vi "_folderExistOrNot_UpData_vna_wmg.vi"(1 "基础路径":path) -> (0 "output":string[](array[string]))   [LabVIEW 2011]
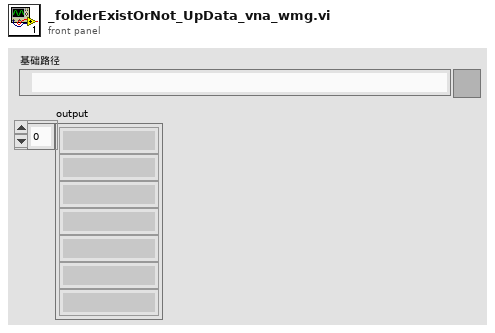
[diagram p1: front panel]
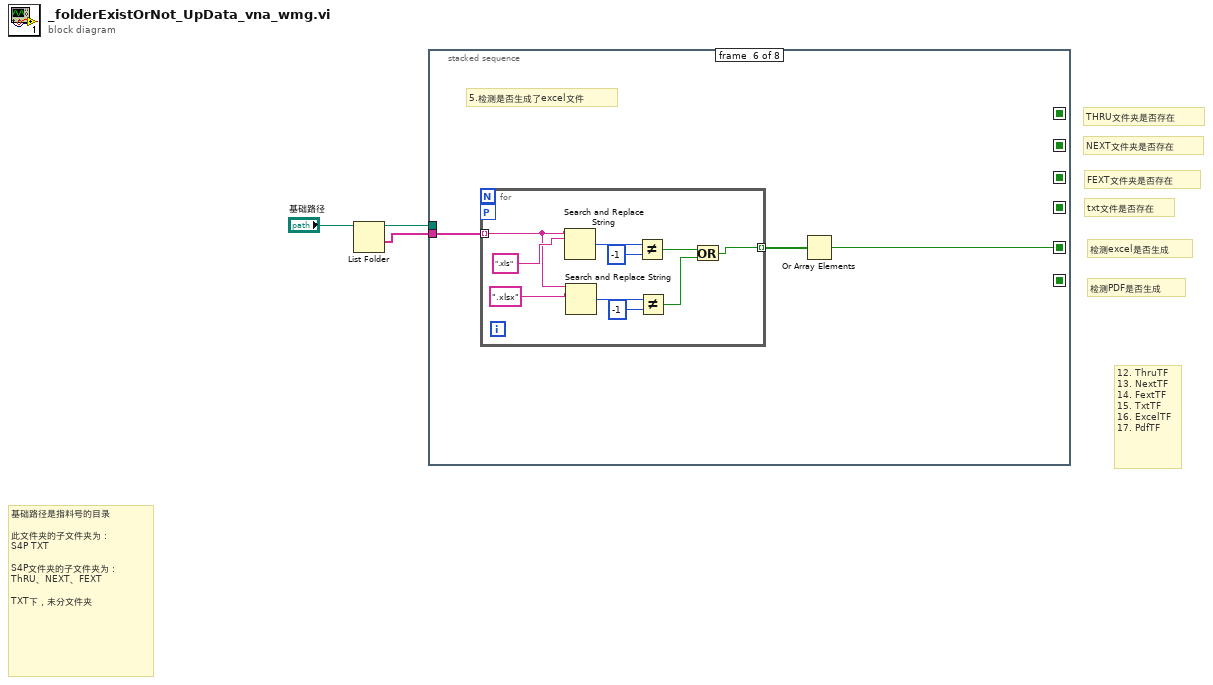
[diagram p0: block diagram]
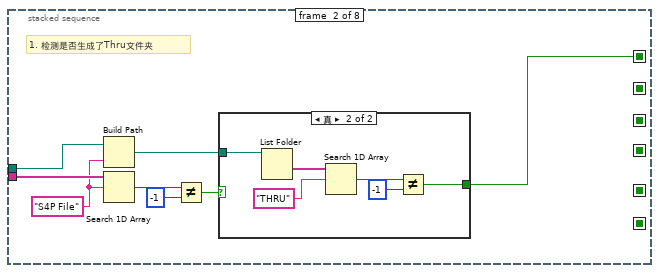
[diagram p3: hidden frame]
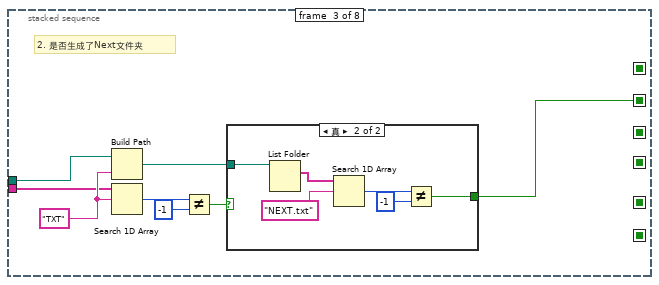
[diagram p5: hidden frame]
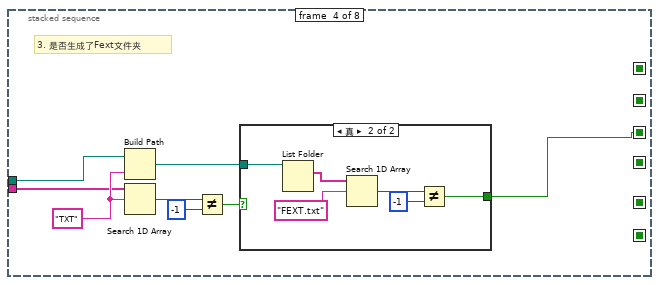
[diagram p7: hidden frame]
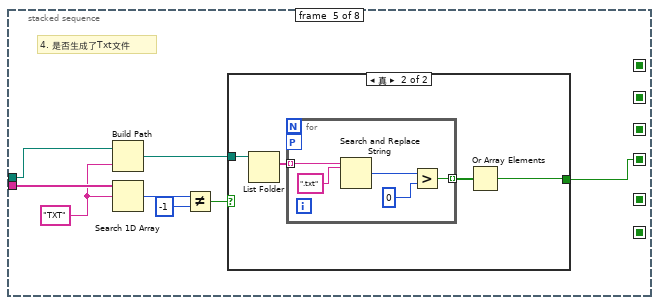
[diagram p9: hidden frame]
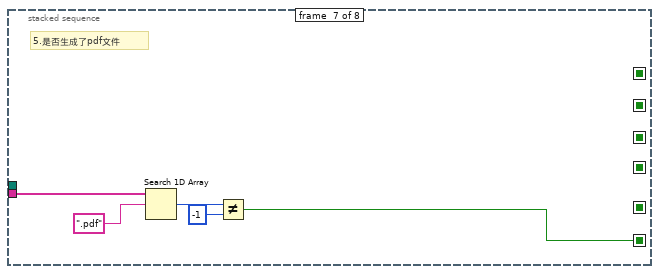
[diagram p11: hidden frame]
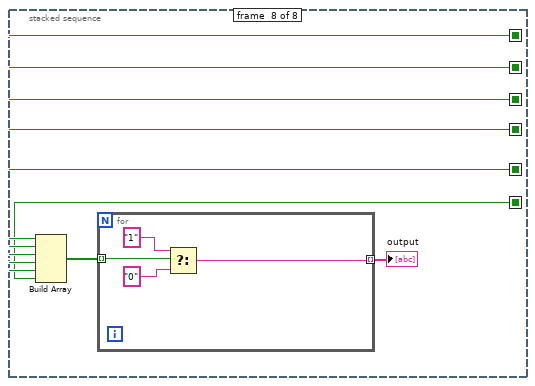
[diagram p12: hidden frame]
diagram:
  # "检测PDF是否生成"
  # "检测excel是否生成"
  # "12. ThruTF\n13. NextTF\n14. FextTF\n15. TxtTF\n16. ExcelTF\n17. PdfTF"
  # "THRU文件夹是否存在"
  # "NEXT文件夹是否存在"
  # "FEXT文件夹是否存在"
  # "txt文件是否存在"
  # "基础路径是指料号的目录\n\n此文件夹的子文件夹为：\nS4P TXT\n\nS4P文件夹的子文件夹为：\nThRU、NEXT、FEXT\n\nTXT下，未分文件夹"
  n1 = List Folder(path="基础路径") -> (path out=w2:path, folder names=w1:string[])  [unwired: 3 in, 2 out]
  n2 = stacked-sequence {
    seq-local: [_ _ _ _ w49 _ _ _] -> [_ _ _ _ _ _ _ w89]
    seq-local: [_ _ _ w34 _ _ _ _] -> [_ _ _ _ _ _ _ w90]
    seq-local: [_ _ w19 _ _ _ _ _] -> [_ _ _ _ _ _ _ w91]
    seq-local: [_ w4 _ _ _ _ _ _] -> [_ _ _ _ _ _ _ w92]
    seq-local: [_ _ _ _ _ w68 _ _] -> [_ _ _ _ _ _ _ w88]
    seq-local: [_ _ _ _ _ _ w80 _] -> [_ _ _ _ _ _ _ w87]
    tunnel: w1 -> [_ w11 w20 w35 w54 w67 w81 _]
    tunnel: w2 -> [_ w7 w21 w36 w52 _ _ _]
    frame #0 {
    }
    frame #1 {
      w6 = "S4P File"
      # "1. 检测是否生成了Thru文件夹"
      n3 = Build Path(base path=w7, name or relative path=w6) -> (appended path=w5:path)
      n4 = Search 1D Array(1D array=w11, element=w6) -> (index of element=w10:i32)  [unwired: 1 in]
      n5 = Not Equal?(x=w10, y=-1) -> (x != y?=w8:bool)
      n6 = case shown="真" w8 {
        selector: w8 -> [w12 _]
        tunnel: w5 -> [_ w15]
        tunnel: [w12 w13] -> w4
        frame False {
        }
        frame True {
          n7 = List Folder(path=w15) -> (folder names=w14:string[])  [unwired: 3 in, 3 out]
          n8 = Search 1D Array(1D array=w14, element="THRU") -> (index of element=w17:i32)  [unwired: 1 in]
          n9 = Not Equal?(x=w17, y=-1) -> (x != y?=w13:bool)
        }
      }
    }
    frame #2 {
      w23 = "TXT"
      # "2. 是否生成了Next文件夹"
      n10 = Build Path(base path=w21, name or relative path=w23) -> (appended path=w22:path)
      n11 = Search 1D Array(1D array=w20, element=w23) -> (index of element=w26:i32)  [unwired: 1 in]
      n12 = Not Equal?(x=w26, y=-1) -> (x != y?=w24:bool)
      n13 = case shown="真" w24 {
        selector: w24 -> [w27 _]
        tunnel: w22 -> [_ w30]
        tunnel: [w27 w29] -> w19
        frame False {
        }
        frame True {
          n14 = List Folder(path=w30) -> (filenames=w28:string[])  [unwired: 3 in, 3 out]
          n15 = Search 1D Array(1D array=w28, element="NEXT.txt") -> (index of element=w32:i32)  [unwired: 1 in]
          n16 = Not Equal?(x=w32, y=-1) -> (x != y?=w29:bool)
        }
      }
    }
    frame #3 {
      w38 = "TXT"
      # "3. 是否生成了Fext文件夹"
      n17 = Build Path(base path=w36, name or relative path=w38) -> (appended path=w37:path)
      n18 = Search 1D Array(1D array=w35, element=w38) -> (index of element=w41:i32)  [unwired: 1 in]
      n19 = Not Equal?(x=w41, y=-1) -> (x != y?=w39:bool)
      n20 = case shown="真" w39 {
        selector: w39 -> [w42 _]
        tunnel: w37 -> [_ w45]
        tunnel: [w42 w44] -> w34
        frame False {
        }
        frame True {
          n21 = List Folder(path=w45) -> (filenames=w43:string[])  [unwired: 3 in, 3 out]
          n22 = Search 1D Array(1D array=w43, element="FEXT.txt") -> (index of element=w47:i32)  [unwired: 1 in]
          n23 = Not Equal?(x=w47, y=-1) -> (x != y?=w44:bool)
        }
      }
    }
    frame #4 {
      w51 = "TXT"
      # "4. 是否生成了Txt文件"
      n24 = Build Path(base path=w52, name or relative path=w51) -> (appended path=w50:path)
      n25 = Search 1D Array(1D array=w54, element=w51) -> (index of element=w56:i32)  [unwired: 1 in]
      n26 = Not Equal?(x=w56, y=-1) -> (x != y?=w53:bool)
      n27 = case shown="真" w53 {
        selector: w53 -> [w57 _]
        tunnel: w50 -> [_ w61]
        tunnel: [w57 w58] -> w49
        frame False {
        }
        frame True {
          n28 = List Folder(path=w61) -> (filenames=w59:string[])  [unwired: 3 in, 3 out]
          n29 = for "For循环" {
            tunnel: [w64] -> w60 mode=indexing
            tunnel: w59 -> [w63] mode=indexing
            workers-P: _ -> [_]
            n30 = Search and Replace String(input string=w63, search string=".txt" ("元素")) -> (number of replacements=w65:i32)  [unwired: 6 in, 3 out]
            n31 = Greater?(x=w65, y=0) -> (0:w64:bool)
          }
          n32 = Or Array Elements(Boolean array=w60) -> (logical OR=w58:bool)
        }
      }
    }
    frame #5 {
      # "5.检测是否生成了excel文件"
      n33 = for "For循环" {
        tunnel: w67 -> [w71] mode=indexing
        tunnel: [w73] -> w69 mode=indexing
        workers-P: _ -> [_]
        n34 = Search and Replace String(input string=w71, search string=".xls") -> (number of replacements=w79:i32)  [unwired: 6 in, 3 out]
        n35 = Search and Replace String(input string=w71, search string=".xlsx") -> (number of replacements=w76:i32)  [unwired: 6 in, 3 out]
        n36 = Not Equal?(x=w79, y=-1) -> (x != y?=w75:bool)
        n37 = Not Equal?(x=w76, y=-1) -> (x != y?=w74:bool)
        n38 = Or(x=w75, y=w74) -> (x .or. y?=w73:bool)
      }
      n39 = Or Array Elements(Boolean array=w69) -> (logical OR=w68:bool)
    }
    frame #6 {
      # "5.是否生成了pdf文件"
      n40 = Search 1D Array(1D array=w81, element=".pdf") -> (index of element=w84:i32)  [unwired: 1 in]
      n41 = Not Equal?(x=w84, y=-1) -> (x != y?=w80:bool)
    }
    frame #7 {
      n42 = Build Array(w92, w91, w90, w89, w88, w87) -> (w86:bool[])
      n43 = for "For循环" {
        tunnel: w86 -> [w96] mode=indexing
        tunnel: [w93] -> w85 mode=indexing
        n44 = Select(t="1", s=w96, f="0") -> (s? t:f=w93:string)
      }
      "output" <- w85
    }
  }
